vi "GUI_laptop v11f.vi"() -> ()   [LabVIEW 2019]
uses:
  <vilib>/Math Plots/3D Math Plots/3D Scatter/3D Scatter XCtrl/3D Scatter.xctl
  <vilib>/Platform/TimedLoop/XDataNode/timing_clust.ctl
  <vilib>/Platform/TimedLoop/XDataNode/nitl_modes.ctl
  <vilib>/Platform/TimedLoop/XDataNode/wakeup.ctl
  <vilib>/Analysis/_algsub.llb/Real Vector Norm.vi
  <vilib>/Instr/_visa.llb/VISA Configure Serial Port (Instr).vi
  <vilib>/Utility/file.llb/Write Delimited Spreadsheet (DBL).vi
  <vilib>/addons/System Identification/Data Preprocess.llb/SI Lowpass Filter (MISO Array).vi
  <vilib>/Math Plots/3D Math Plots/3D Scatter/3D Scatter Datatype/Public/Plot Helper (Vector).vi
  <vilib>/platform/TimedLoop/XDataNode/XDataNode.xnode
  <vilib>/Platform/TimedLoop/XDataNode/XDNodeRunTimeDep.lvlib
  <vilib>/Analysis/NI_AALPro.lvlib
  <vilib>/Math Plots/3D Math Plots/3D Scatter/3D Scatter Datatype/3D Scatter Datatype.lvclass
  <vilib>/addons/System Identification/NI_SysID.lvlib
panel:
  in  "Sample rate":u32=115200
  in  "Cutoff Frequency":dbl=10.0
  in  "Motion scale L1 L2":dbl=10.0
  in  "Motion scale L3":dbl=2.0
  in  "Save Path 4":path=path "C:/Users/jimmy/Documents/GitHub/Arduino-LabVIEW/zhantao/read_data_abs_filtered.csv"
  in  "Save Path 3":path=path "C:/Users/jimmy/Documents/GitHub/Arduino-LabVIEW/zhantao/read_data_abs_sending.csv"
  out "stimulus signals out":dbl[][](array[numeric]) format="%.2f"
  in  "L5 Offset":dbl
  in  "L5 Scale":dbl=1.0
  in  "Motion Scale L4":dbl=2.0
  out "spreadsheet string":string
  in  "Save Path 2":path=path "C:/Users/jimmy/Documents/GitHub/Arduino-LabVIEW/zhantao/read_data_delt.csv"
  out "send values":dbl[](array[numeric])
  out "Robot Feedback (xyz)":dbl[](array[numeric])
  in  "UDP Send":bool
  in  "UDP Recv":bool
  in  "L5 bound":dbl=1000.0
  in  "L4 bound (deg)":dbl=1000.0
  in  "L3 bound (mm)":dbl=1000.0
  in  "L2 bound (deg)":dbl=1000.0
  in  "L1 bound (deg)":dbl=1000.0
  in  "Joystick Type":dbl(ring) items=["Rigid Joystick", "Free Joystick"]
  out "Finished Late? [i-1]":bool
  in  "Epsilon":dbl=0.2
  out "3D Scatter":refnum<class "3D Plot Datatype.lvclass">[](xcontrol)
  out "Random Point":dbl[](array[numeric])
  out "Virtual Cursor":dbl[](array[numeric])
  out "Iteration Duration":i64
  in  "Num of Points":i32=10
  in  "z bound":dbl=2.0
  in  "y bound":dbl=5.0
  in  "x bound":dbl=5.0
  in  "Stop":bool
  in  "Round Decimals":dbl=2.0 format="%#_15g"
  in  "Save Data":bool
  in  "Save Path":path=path "C:/Users/jimmy/Documents/GitHub/Arduino-LabVIEW/zhantao/read_data_abs.csv"
  in  "x speed":dbl=0.5
  in  "z speed":dbl=0.5
  in  "y speed":dbl=0.5
  out "error out":errorcluster
  in  "baud rate":u32=115200
  in  "VISA resource name":refnum<visa-resource-name>
  # "Joystick Selection"
  # "Plotting"
  # "Data Saving"
  # "Arduino Communication"
  # "Master Slave Communication"
  # "Parameters"
  # "TODO: fix the bounds; currently bounds are arbitrary"
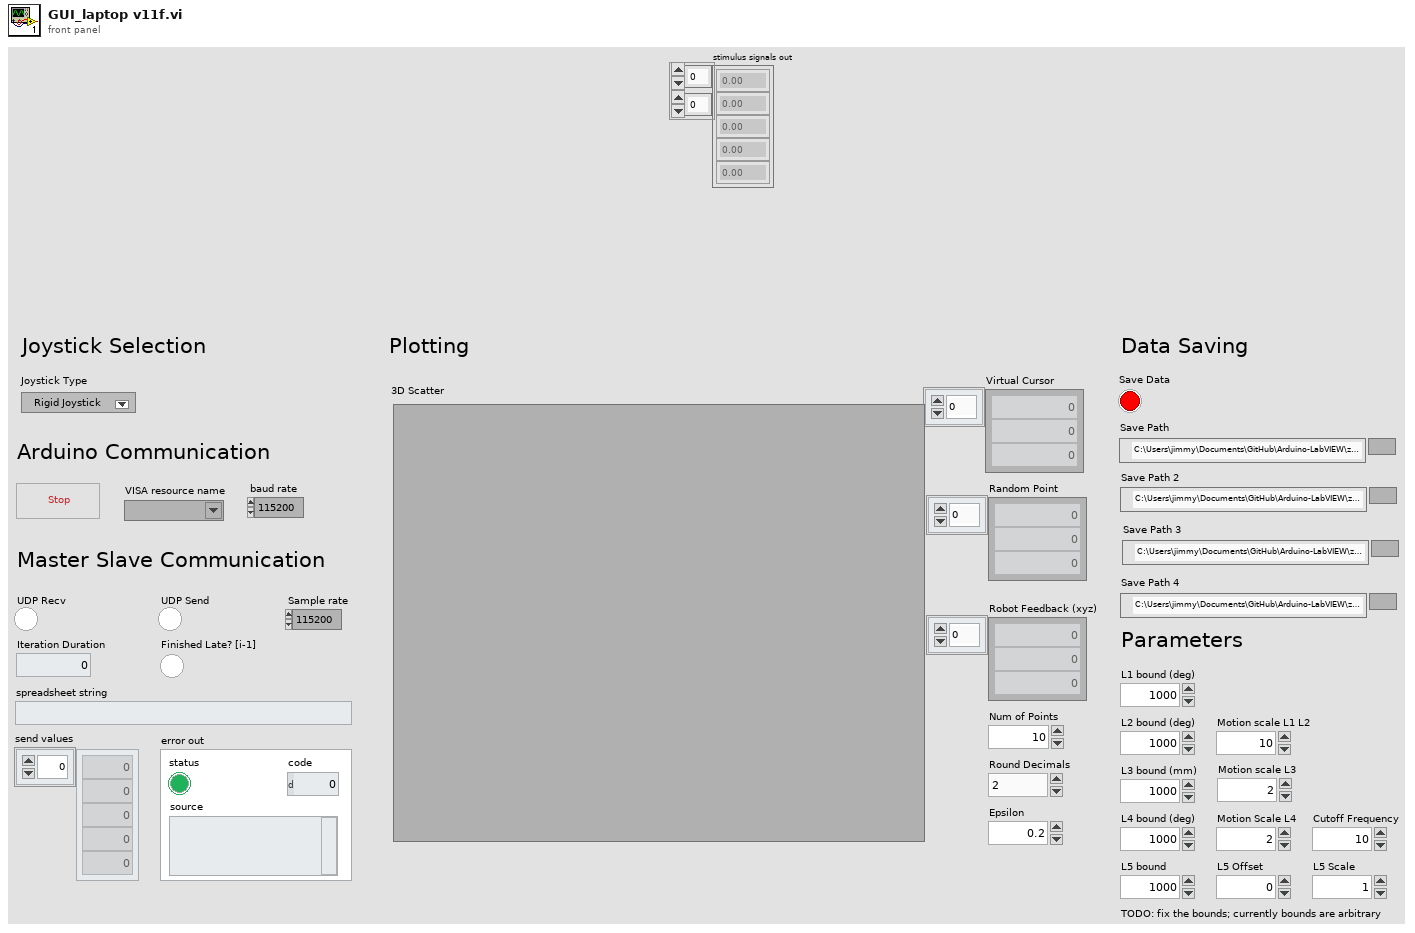
[diagram p1: front panel]
types:
  T1 = typedef "XDNodeRunTimeDep.lvlib/timing_clust.ctl" = cluster{"Expected End [f-1]":u64, "Actual End [f-1]":u64, "Finished Late? [f-1]":bool, "Expected End [i-1]":u64, "Actual End [i-1]":u64, "Finished Late? [i-1]":bool, "Expected Start [i]":u64, "Actual Start [i]":u64, "Expected Start [f]":u64, "Actual Start [f]":u64, "Source Name":string, "Structure Name":string, "Period":i64, "Deadline":i64, "Offset":i64, "Start":i64, "Priority":i32, "Timeout":i32, "Mode":T2, "Wakeup Reason":T3, "Error":errorcluster, "Source Type":string, "Secondary Source Type":string, "Global End Time":u64, "Global Start Time":u64, "Frame Duration":u64, "Iteration Duration":u64, "Assigned CPU":i32, "I/O Scan Engine Mode":u32}
  T2 = typedef "XDNodeRunTimeDep.lvlib/nitl_modes.ctl" = enum32{"No Change", "Process missed periods, maintain original phase", "Discard missed periods, maintain original phase", "Process missed periods, ignore original phase", "Discard missed periods, ignore original phase"}
  T3 = typedef "XDNodeRunTimeDep.lvlib/wakeup.ctl" = enum32{"Normal", "Aborted", "Asynchronous wakeup", "Timing source error", "Timed loop error", "Timeout"}
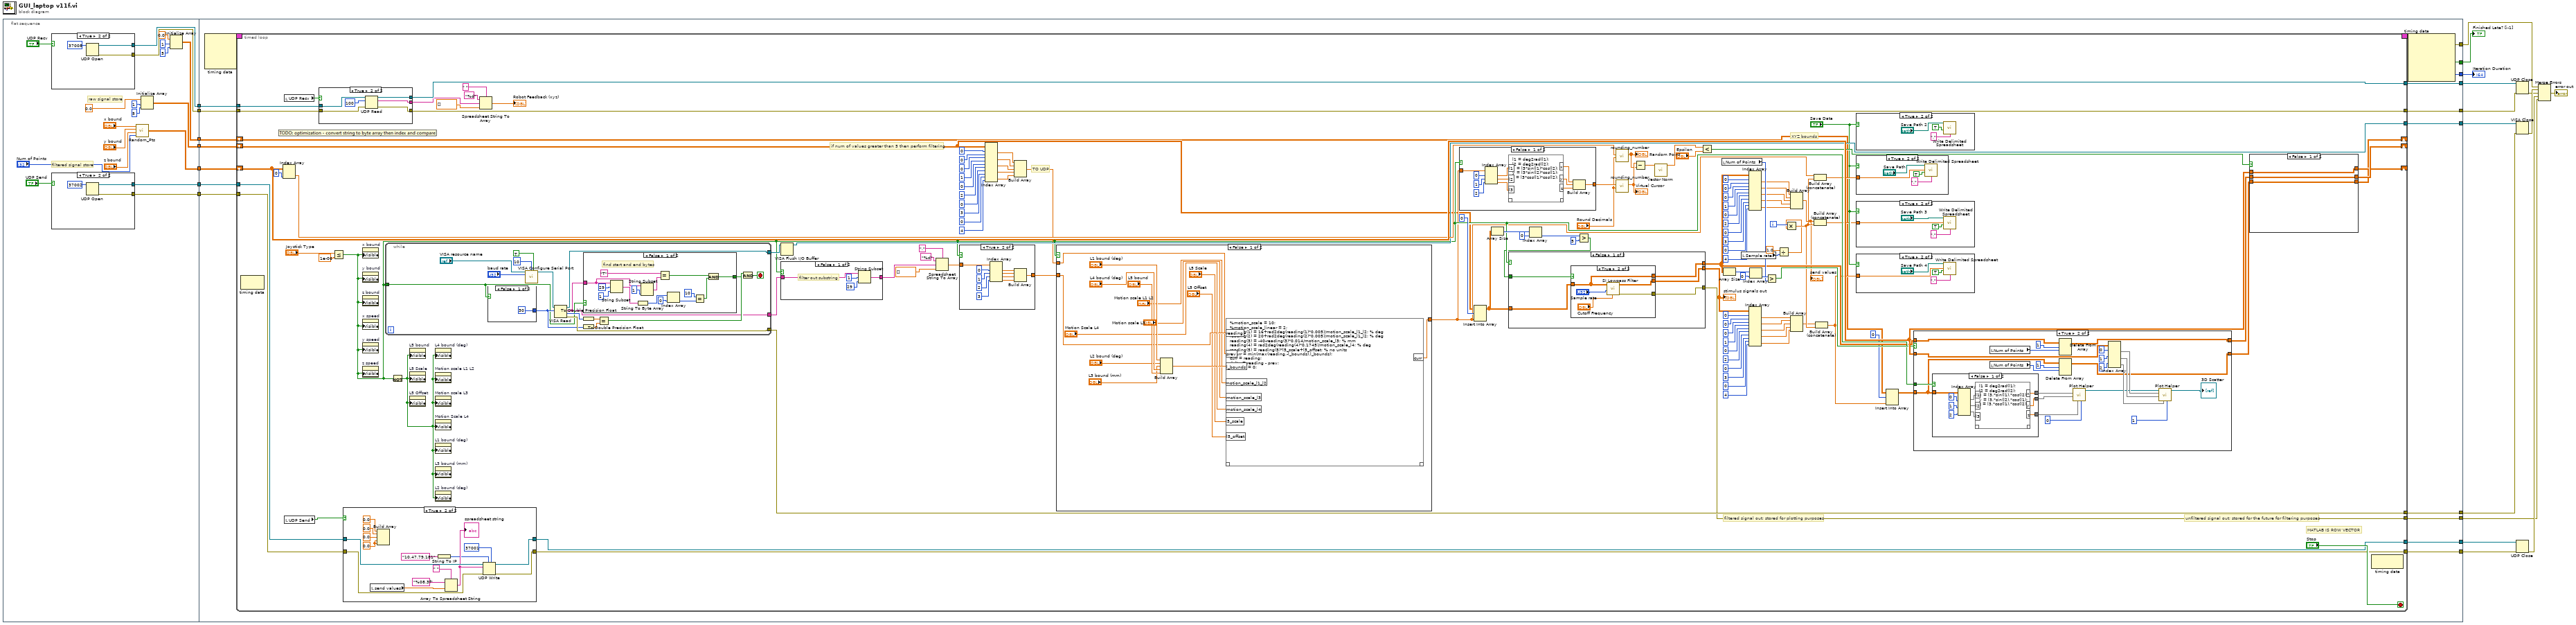
[diagram p0: block diagram]
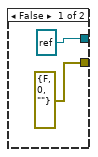
[diagram p2: hidden frame]
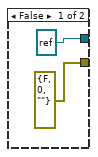
[diagram p3: hidden frame]
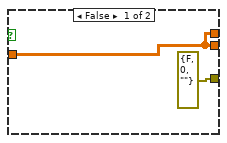
[diagram p6: hidden frame]
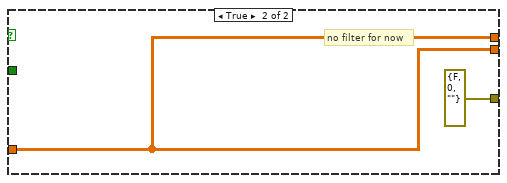
[diagram p7: hidden frame]
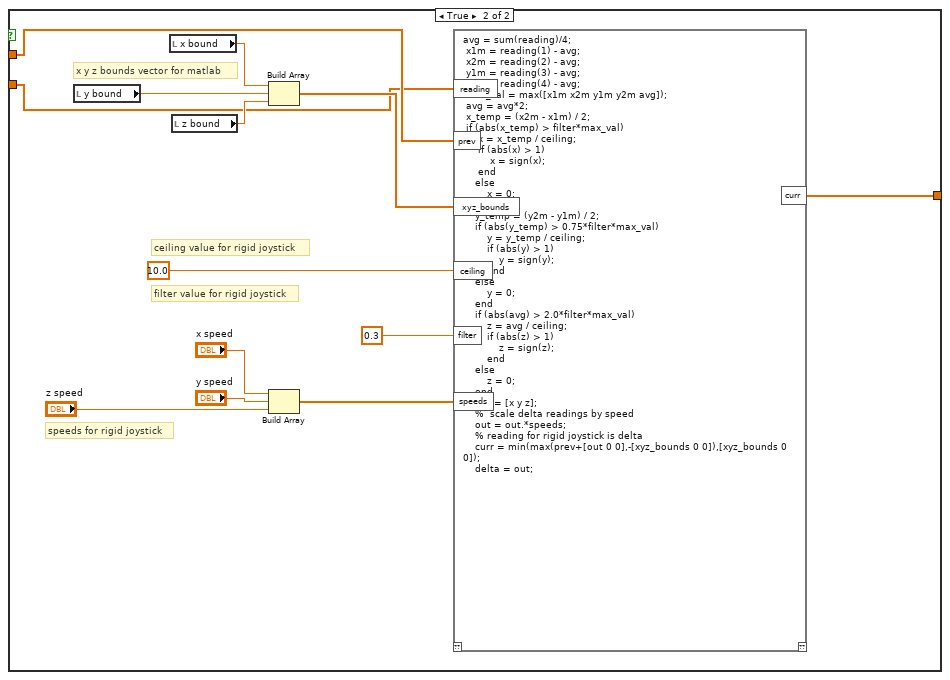
[diagram p8: hidden frame]
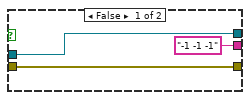
[diagram p11: hidden frame]
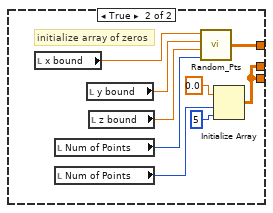
[diagram p13: hidden frame]
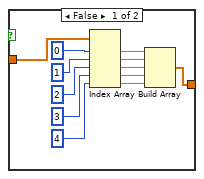
[diagram p15: hidden frame]
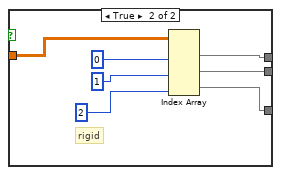
[diagram p18: hidden frame]
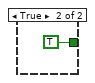
[diagram p19: hidden frame]
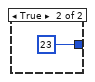
[diagram p20: hidden frame]
diagram:
  n1 = flat-sequence {
    tunnel: [w32] -> w17
    tunnel: [w36] -> w16
    tunnel: [w31] -> w15
    tunnel: [w30] -> w14
    tunnel: [w27] -> w13
    tunnel: [w26] -> w12
    tunnel: [w22] -> w1
    tunnel: [w67] -> w21
    tunnel: [w66] -> w20
    tunnel: [w64] -> w11
    tunnel: [w62] -> w19
    tunnel: [w61] -> w18
    tunnel: w17 -> [w65]
    tunnel: w16 -> [w63]
    tunnel: w15 -> [w60]
    tunnel: w14 -> [w59]
    tunnel: w13 -> [w58]
    tunnel: w12 -> [w57]
    tunnel: [w56] -> w5
    tunnel: [w55] -> w10
    tunnel: [w54] -> w4
    tunnel: [w53] -> w3
    tunnel: [w52] -> w2
    tunnel: w1 -> [w51]
    frame #0 {
      # "filtered signal store"
      # "raw signal store"
      n2 = case shown="True" "UDP Recv" {
        tunnel: [refnum<k16> refnum ("port") w49] -> w30
        tunnel: [errorcluster {"status"=FALSE, "code"=0, "source"=""} ("error out") w48] -> w27
        frame False {
        }
        frame True {
          n3 = UDP Open(11:u16 37008 ("port")) -> (port=w49:refnum<k16>, 0:w48:errorcluster)  [unwired: 4 in, 1 out]
        }
      }
      n4 = case shown="True" "UDP Send" {
        tunnel: [refnum<k16> refnum ("port") w44] -> w31
        tunnel: [errorcluster {"status"=FALSE, "code"=0, "source"=""} ("error out") w43] -> w26
        frame False {
        }
        frame True {
          n5 = UDP Open(11:u16 37002 ("port")) -> (port=w44:refnum<k16>, 0:w43:errorcluster)  [unwired: 4 in, 1 out]
        }
      }
      n6 = call "Random_Pts.vi"("Num of Points"="Num of Points", "z bound"="z bound", "y bound"="y bound", "x bound"="x bound") -> ("appended array"=w36:dbl[][])
      n7 = Initialize Array(0.0 ("element"), 1 ("dimension size"), 5 ("dimension size")) -> (w32:dbl[][])
      n8 = Initialize Array(0.0 ("element"), 1 ("dimension size"), 5 ("dimension size")) -> (w22:dbl[][])
    }
    frame #1 {
      n9 = node-c288() -> (w69:T1)  [unwired: 4 in]
      n10 = timed-loop {
        tunnel: [w134] -> w67
        tunnel: [w191] -> w66
        shift-right: [w190] -> _
        shift-left: w65 -> [w88]
        timing: w69 -> [_]
        timing-out: [_] -> w68
        shift-right: [w186] -> _
        shift-left: w63 -> [w187]
        tunnel: w60 -> [w149]
        tunnel: w59 -> [w148]
        tunnel: w58 -> [w146]
        tunnel: w57 -> [w145]
        tunnel: [w144] -> w56
        tunnel: [w143] -> w55
        tunnel: [w142] -> w54
        tunnel: [w141] -> w53
        tunnel: [w123] -> w52
        shift-right: [w79] -> _
        shift-left: w51 -> [w82]
        i -> [w77]
        stop <- "Stop" stop-if-true
        # "unfiltered signal out; stored for the future for filtering purposes"
        # "filtered signal out; stored for plotting purposes"
        # "XYZ bounds"
        # "if num of values greater than 5 then perform filtering"
        # "TO UDP"
        # "MATLAB IS ROW VECTOR"
        n11 = node-c288() -> ()  [unwired: 1 in, 1 out]
        n12 = Index Array(array=w187, index (col)=0 ("index (row)")) -> (element=w158:dbl[])  [unwired: 1 in]
        n13 = local read "UDP Recv"() -> (w147:bool)
        n14 = local read "UDP Send"() -> (w72:bool)
        n15 = case shown="True" w147 {
          tunnel: w148 -> [w263 w270]
          tunnel: w146 -> [w264 w269]
          tunnel: [w264 w268] -> w144
          tunnel: [w263 w267] -> w142
          tunnel: ["-1 -1 -1" w265] -> w137
          frame False {
          }
          frame True {
            n16 = UDP Read(connection ID=w270, max size (548)=100, 8:w269) -> (data out=w265:string, error out=w268:errorcluster, 3:w267:refnum<k16>)  [unwired: 1 in, 2 out]
          }
        }
        n17 = Less Or Equal?(x="Joystick Type", y=1e-06) -> (x <= y?=w124:bool)
        n18 = case shown="True" w72 {
          tunnel: w149 -> [w245 w261]
          tunnel: w145 -> [w246 w257]
          tunnel: [w246 w253] -> w143
          tunnel: [w245 w252] -> w141
          frame False {
          }
          frame True {
            w251 = 0.0 ("element")
            n19 = local read "send values"() -> (w247:dbl[])
            n20 = Build Array(0.0 ("element"), 0.0 ("element"), 0.0 ("element"), w251, w251) -> ()  [unwired: 1 out]
            n21 = String To IP(1:"10.47.79.181" ("name")) -> (0:w255:u32)
            n22 = Array To Spreadsheet String(delimiter (Tab)=" ", array=w247, 3:"%08.3f" ("format string")) -> (spreadsheet string=w258:string)
            "spreadsheet string" <- w258
            n23 = UDP Write(address=w255, port or service name=u16 37001, connection ID=w261, data in=w258, 8:w257) -> (error out=w253:errorcluster, 3:w252:refnum<k16>)  [unwired: 1 in]
          }
        }
        n24 = property on="x bound" class="DigNum (strict)"("Visible"=w124) -> ()  [unwired: 2 in, 2 out]
        n25 = property on="y bound" class="DigNum (strict)"("Visible"=w124) -> ()  [unwired: 2 in, 2 out]
        n26 = property on="z bound" class="DigNum (strict)"("Visible"=w124) -> ()  [unwired: 2 in, 2 out]
        n27 = property on="x speed" class="DigNum (strict)"("Visible"=w124) -> ()  [unwired: 2 in, 2 out]
        n28 = property on="y speed" class="DigNum (strict)"("Visible"=w124) -> ()  [unwired: 2 in, 2 out]
        n29 = property on="z speed" class="DigNum (strict)"("Visible"=w124) -> ()  [unwired: 2 in, 2 out]
        n30 = while {
          tunnel: [w368] -> w160
          tunnel: [w381] -> w191
          tunnel: [w375] -> w135
          tunnel: w124 -> [w369]
          stop <- w371 stop-if-true
          n31 = case shown="False" w369 {
            tunnel: [30 u32 23 ("byte count")] -> w374
            frame False {
            }
            frame True {
            }
          }
          n32 = call-poly "VISA Configure Serial Port"("VISA resource name"="VISA resource name", "termination char\n(0xA = '\\n' = LF)"=u8 10 ("termination char\n(0xA = '\\n' = LF)"), "Enable Termination\nChar (T)"=TRUE ("Enable Termination\nChar (T)"), "baud rate (9600)"="baud rate") -> ("VISA resource name out"=w376:refnum<visa-resource-name>)  [unwired: 10 in, 1 out]
          n33 = VISA Read(VISA resource name=w376, byte count=w374) -> (VISA resource name out=w375:refnum<visa-resource-name>, read buffer=w368:string, return count=w383:u32, error out=w381:errorcluster)  [unwired: 1 in]
          n34 = To Double Precision Float(number=w383) -> (double precision float=w382:dbl)
          n35 = To Double Precision Float(number=w374) -> (double precision float=w373:dbl)
          n36 = case shown="False" w369 {
            tunnel: [w390 TRUE] -> w370
            tunnel: w368 -> [w393 _]
            frame False {
              # "find start and end bytes"
              n37 = String Subset(string=w393, offset (0)=29, length (rest)=1) -> (substring=w388:string)
              n38 = String To Byte Array(string=w388) -> (unsigned byte array=w387:u8[])
              n39 = String Subset(string=w393, length (rest)=1) -> (substring=w396:string)  [unwired: 1 in]
              n40 = Equal?(x="T", y=w396) -> (x = y?=w392:bool)
              n41 = Index Array(array=w387, index=0) -> (element=w385:u8)
              n42 = Equal?(x=10, y=w385) -> (x = y?=w391:bool)
              n43 = And(x=w392, y=w391) -> (x .and. y?=w390:bool)
            }
            frame True {
            }
          }
          n44 = Equal?(x=w382, y=w373) -> (x = y?=w372:bool)
          n45 = And(x=w372, y=w370) -> (x .and. y?=w371:bool)
        }
        n46 = Not(x=w124) -> (.not. x?=w86:bool)
        n47 = property on="L5 bound" class="DigNum (strict)"("Visible"=w86) -> ()  [unwired: 2 in, 2 out]
        n48 = property on="L5 Scale" class="DigNum (strict)"("Visible"=w86) -> ()  [unwired: 2 in, 2 out]
        n49 = property on="L5 Offset" class="DigNum (strict)"("Visible"=w86) -> ()  [unwired: 2 in, 2 out]
        n50 = property on="L4 bound (deg)" class="DigNum (strict)"("Visible"=w86) -> ()  [unwired: 2 in, 2 out]
        n51 = property on="Motion scale L1 L2" class="DigNum (strict)"("Visible"=w86) -> ()  [unwired: 2 in, 2 out]
        n52 = property on="Motion scale L3" class="DigNum (strict)"("Visible"=w86) -> ()  [unwired: 2 in, 2 out]
        n53 = property on="Motion Scale L4" class="DigNum (strict)"("Visible"=w86) -> ()  [unwired: 2 in, 2 out]
        n54 = property on="L1 bound (deg)" class="DigNum (strict)"("Visible"=w86) -> ()  [unwired: 2 in, 2 out]
        n55 = property on="L3 bound (mm)" class="DigNum (strict)"("Visible"=w86) -> ()  [unwired: 2 in, 2 out]
        n56 = property on="L2 bound (deg)" class="DigNum (strict)"("Visible"=w86) -> ()  [unwired: 2 in, 2 out]
        n57 = Spreadsheet String To Array(delimiter (Tab)=" ", format string="%d", spreadsheet string=w137, array type (2D Dbl)=dbl[] []) -> (array=→"Robot Feedback (xyz)":dbl[])
        n58 = VISA Flush I/O Buffer(VISA resource name=w135) -> (VISA resource name out=w134:refnum<visa-resource-name>)  [unwired: 2 in, 1 out]
        n59 = case shown="False" w124 {
          tunnel: w160 -> [w290 w291]
          tunnel: [w287 w291] -> w159
          frame False {
            # "filter out substring"
            n60 = String Subset(string=w290, offset (0)=1, length (rest)=29) -> (substring=w287:string)
          }
          frame True {
          }
        }
        n61 = Spreadsheet String To Array(delimiter (Tab)=",", format string="%d", spreadsheet string=w159, array type (2D Dbl)=dbl[] []) -> (array=w161:dbl[])
        n62 = case shown="True" w124 {
          tunnel: w161 -> [w292 w307]
          tunnel: [w297 w306] -> w132
          frame False {
            n63 = Index Array(array=w292, index #1=0 ("Plot ID"), index #2=1 ("Plot ID"), index #3=2 ("Plot ID"), index #4=3 ("Plot ID"), index #5=4 ("Plot ID")) -> (element #1=w300:dbl, element #2=w299:dbl, element #3=w298:dbl, element #4=w294:dbl, element #5=w293:dbl)
            n64 = Build Array(w300, w299, w298, w294, w293) -> (w297:dbl[])
          }
          frame True {
            n65 = Index Array(array=w307, index #1=0 ("Plot ID"), index #2=1 ("Plot ID"), index #3=2 ("Plot ID"), index #4=3 ("index")) -> (element #1=w310:dbl, element #2=w309:dbl, element #3=w308:dbl, element #4=w304:dbl)
            n66 = Build Array(w310, w309, w308, w304) -> (w306:dbl[])
          }
        }
        n67 = Index Array(array=w88, index (row) #1=0 ("disabled index (row)"), index (col) #1=0 ("disabled index (col)"), index (row) #2=0 ("disabled index (row)"), index (col) #2=1 ("disabled index (col)"), index (row) #3=0 ("disabled index (row)"), index (col) #3=2 ("disabled index (col)"), index (row) #4=0 ("disabled index (row)"), index (col) #4=3 ("disabled index (col)"), index (row) #5=0 ("disabled index (row)"), index (col) #5=4 ("disabled index (col)")) -> (element #1=w172:dbl, element #2=w171:dbl, element #3=w170:dbl, element #4=w163:dbl, element #5=w162:dbl)
        n68 = Build Array(w172, w171, w170, w163, w162) -> (w133:dbl[])
        n69 = case shown="False" w124 {
          tunnel: w133 -> [w220 w231]
          tunnel: w132 -> [w221 w230]
          tunnel: [w219 w229] -> w107
          frame False {
            n70 = Build Array("L1 bound (deg)", "L2 bound (deg)", "L3 bound (mm)", "L4 bound (deg)", "L5 bound") -> (w222:dbl[])
            n71 = script code="%motion_scale = 10;\n%motion_scale_linear = 2;\nreading(1) = 16+rad2deg(reading(1)*0.005)/motion_scale_l1_l2; % deg\nreading(2) = 20+rad2deg(reading(2)*0.005)/motion_scale_l1_l2; % deg\nreading(3) = -40-reading(3)*0.014/motion_scale_l3; % mm\nreading(4) = rad2deg(reading(4)*0.1745)/motion_scale_l4; % deg\nreading(5) = reading(5)*l5_scale+l5_offset; % no units\n%curr = min(max(reading,-l_bounds),l_bounds);\ncurr = reading;\ndelta = reading - prev;\ndelta(5) = 0;"("l_bounds"=w222, "motion_scale_l4"="Motion Scale L4", "reading"=w221, "prev"=w220, "l5_scale"="L5 Scale", "l5_offset"="L5 Offset", "motion_scale_l3"="Motion scale L3", "motion_scale_l1_l2"="Motion scale L1 L2") -> ("curr"=w219:dbl[])  [unwired: 1 in, 1 out]
          }
          frame True {
            # "ceiling value for rigid joystick"
            # "filter value for rigid joystick"
            # "speeds for rigid joystick"
            # "x y z bounds vector for matlab"
            n72 = local read "y bound"() -> (w240:dbl)
            n73 = local read "x bound"() -> (w239:dbl)
            n74 = local read "z bound"() -> (w241:dbl)
            n75 = Build Array(w239, w240, w241) -> (w232:dbl[])
            n76 = Build Array("x speed", "y speed", "z speed") -> (w235:dbl[])
            n77 = script code="avg = sum(reading)/4;\n x1m = reading(1) - avg;\n x2m = reading(2) - avg;\n y1m = reading(3) - avg;\n y2m = reading(4) - avg;\n max_val = max([x1m x2m y1m y2m avg]);\n avg = avg*2;\n x_temp = (x2m - x1m) / 2;\n if (abs(x_temp) > filter*max_val)\n     x = x_temp / ceiling;\n     if (abs(x) > 1)\n         x = sign(x);\n     end\n    else\n        x = 0;\n    end\n    y_temp = (y2m - y1m) / 2;\n    if (abs(y_temp) > 0.75*filter*max_val)\n        y = y_temp / ceiling;\n        if (abs(y) > 1)\n            y = sign(y);\n        end\n    else\n        y = 0;\n    end\n    if (abs(avg) > 2.0*filter*max_val)\n        z = avg / ceiling;\n        if (abs(z) > 1)\n            z = sign(z);\n        end\n    else\n        z = 0;\n    end\n    out = [x y z];\n    %  scale delta readings by speed\n    out = out.*speeds;\n    % reading for rigid joystick is delta\n    curr = min(max(prev+[out 0 0],-[xyz_bounds 0 0]),[xyz_bounds 0 0]);\n    delta = out;"("xyz_bounds"=w232, "ceiling"=10.0 ("Real"), "filter"=0.3 ("Real"), "speeds"=w235, "reading"=w230, "prev"=w231) -> ("curr"=w229:dbl[])  [unwired: 1 in, 1 out]
          }
        }
        n78 = case shown="False" w124 {
          tunnel: [w318 w325] -> w188
          tunnel: w107 -> [w317 w325]
          frame False {
            n79 = Index Array(array=w317, index #1=0 ("Plot ID"), index #2=1 ("Plot ID"), index #3=2 ("Plot ID")) -> (element #1=w316:dbl, element #2=w315:dbl, element #3=w314:dbl)
            n80 = script code="l1 = deg2rad(l1);\nl2 = deg2rad(l2);\nx = l3*sin(l1)*cos(l2);\ny = l3*sin(l2)*cos(l1);\nz = l3*cos(l1)*cos(l2);"("l1"=w316, "l2"=w315, "l3"=w314) -> ("x"=w321:dbl, "y"=w320:dbl, "z"=w319:dbl)  [unwired: 1 in, 1 out]
            n81 = Build Array(w321, w320, w319) -> (w318:dbl[])
          }
          frame True {
          }
        }
        n82 = Insert Into Array(array=w88, index (row)=0, new element=w107) -> (w125:dbl[][])  [unwired: 1 in]
        n83 = Array Size(array=w125) -> (size(s)=w128:i32[])
        n84 = Index Array(array=w128, index=0) -> (element=w127:i32)
        n85 = Greater?(x=w127, y=5) -> (0:w73:bool)
        n86 = case shown="False" w124 {
          tunnel: w73 -> [w203 _]
          tunnel: w125 -> [w205 w213]
          tunnel: [w204 w213] -> w85
          tunnel: [w202 errorcluster {"status"=FALSE, "code"=0, "source"=""} ("error out")] -> w123
          tunnel: [w201 w213] -> w89
          frame False {
            n87 = case shown="True" w203 {
              tunnel: w205 -> [w206 w211]
              tunnel: [w206 w211] -> w204
              tunnel: [errorcluster {"status"=FALSE, "code"=0, "source"=""} ("error out") w212] -> w202
              tunnel: [w206 w210] -> w201
              frame False {
              }
              frame True {
                n88 = call-poly <vilib>:"SI Lowpass Filter.vi"("cutoff frequency"="Cutoff Frequency", "sampling rate (Hz)"="Sample rate", "stimulus signals in"=w211) -> ("error out"=w212:errorcluster, "stimulus signals out"=w210:dbl[][])  [unwired: 6 in, 1 out]
              }
            }
          }
          frame True {
            # "no filter for now"
          }
        }
        "stimulus signals out" <- w89
        n89 = call "rounding_number.vi"("power of ten"="Round Decimals", "Array"=w158) -> ("rounded"=w155:dbl[])  [unwired: 9 in]
        "Random Point" <- w155
        n90 = call "rounding_number.vi"("power of ten"="Round Decimals", "Array"=w188) -> ("rounded"=w156:dbl[])  [unwired: 9 in]
        "Virtual Cursor" <- w156
        n91 = Subtract(x=w156, y=w155) -> (x-y=w154:dbl[])
        n92 = call-poly <vilib>:"Vector Norm.vi"("Input Vector"=w154) -> ("norm"=w153:dbl)  [unwired: 9 in, 1 out]
        n93 = Less?(x=w153, y="Epsilon") -> (x < y?=w151:bool)
        n94 = local read "Num of Points"() -> (w174:i32)
        n95 = Array Size(array=w85) -> (size(s)=w131:i32[])
        n96 = local read "Sample rate"() -> (w74:u32)
        n97 = Index Array(array=w85, index (row) #1=0 ("disabled index (col)"), index (col) #1=0 ("disabled index (row)"), index (row) #2=0 ("disabled index (col)"), index (col) #2=1 ("disabled index (row)"), index (row) #3=0 ("disabled index (col)"), index (col) #3=2 ("disabled index (row)"), index (row) #4=0 ("disabled index (col)"), index (col) #4=3 ("disabled index (row)"), index (row) #5=0 ("disabled index (col)"), index (col) #5=4 ("disabled index (col)")) -> (element #1=w112:dbl, element #2=w111:dbl, element #3=w110:dbl, element #4=w109:dbl, element #5=w108:dbl)
        n98 = Index Array(array=w89, index (row) #1=0 ("disabled index (col)"), index (col) #1=0 ("disabled index (row)"), index (row) #2=0 ("disabled index (col)"), index (col) #2=1 ("disabled index (row)"), index (row) #3=0 ("disabled index (col)"), index (col) #3=2 ("disabled index (row)"), index (row) #4=0 ("disabled index (col)"), index (col) #4=3 ("disabled index (row)"), index (row) #5=0 ("disabled index (col)"), index (col) #5=4 ("disabled index (col)")) -> (element #1=w95:dbl, element #2=w94:dbl, element #3=w93:dbl, element #4=w92:dbl, element #5=w91:dbl)
        n99 = Index Array(array=w131, index=0) -> (element=w175:i32)
        n100 = Greater?(x=w175, y=w174) -> (0:w173:bool)
        n101 = Divide(x=1.0, y=w74) -> (x/y=w75:dbl)
        n102 = Multiply(x=w77, y=w75) -> (x*y=w78:dbl)
        n103 = Build Array(w112, w111, w110, w109, w108) -> (w70:dbl[])
        "send values" <- w70
        n104 = Build Array(w95, w94, w93, w92, w91) -> (w71:dbl[])
        n105 = Build Array (concatenate)(w107, w78) -> (w106:dbl[])
        n106 = Build Array (concatenate)(w70, w78) -> (w87:dbl[])
        n107 = Build Array (concatenate)(w71, w78) -> (w83:dbl[])
        n108 = case shown="True" "Save Data" {
          frame False {
          }
          frame True {
            n109 = call-poly <vilib>:"Write Delimited Spreadsheet.vi"("file path (dialog if empty)"="Save Path 2", "append to file? (new file:F)"=TRUE, "delimiter (\\t)"="," ("delimiter (\\t)")) -> ()  [unwired: 11 in, 2 out]
          }
        }
        n110 = case shown="True" "Save Data" {
          tunnel: w106 -> [_ w271]
          frame False {
          }
          frame True {
            n111 = call-poly <vilib>:"Write Delimited Spreadsheet.vi"("file path (dialog if empty)"="Save Path", "1D data"=w271, "append to file? (new file:F)"=TRUE, "delimiter (\\t)"="," ("delimiter (\\t)")) -> ()  [unwired: 10 in, 2 out]
          }
        }
        n112 = case shown="True" "Save Data" {
          tunnel: w87 -> [_ w197]
          frame False {
          }
          frame True {
            n113 = call-poly <vilib>:"Write Delimited Spreadsheet.vi"("file path (dialog if empty)"="Save Path 3", "1D data"=w197, "append to file? (new file:F)"=TRUE, "delimiter (\\t)"="," ("delimiter (\\t)")) -> ()  [unwired: 10 in, 2 out]
          }
        }
        n114 = case shown="True" "Save Data" {
          tunnel: w83 -> [_ w193]
          frame False {
          }
          frame True {
            n115 = call-poly <vilib>:"Write Delimited Spreadsheet.vi"("file path (dialog if empty)"="Save Path 4", "1D data"=w193, "append to file? (new file:F)"=TRUE, "delimiter (\\t)"="," ("delimiter (\\t)")) -> ()  [unwired: 10 in, 2 out]
          }
        }
        n116 = Insert Into Array(array=w82, index (row)=0, new element=w83) -> (w81:dbl[][])  [unwired: 1 in]
        n117 = case shown="True" w173 {
          tunnel: w85 -> [w327 w349]
          tunnel: [w327 w348] -> w189
          tunnel: w187 -> [w326 w347]
          tunnel: w124 -> [_ w332]
          tunnel: w81 -> [_ w329]
          tunnel: [w326 w328] -> w80
          frame False {
          }
          frame True {
            n118 = case shown="False" w332 {
              tunnel: w329 -> [w360 w364]
              tunnel: [w351 w363] -> w338
              tunnel: [w352 w362] -> w337
              tunnel: [w353 w361] -> w336
              frame False {
                n119 = Index Array(array=w360, index (col) #1=0 ("Plot ID"), index (col) #2=1 ("Plot ID"), index (col) #3=2 ("Plot ID")) -> (element #1=w356:dbl[], element #2=w355:dbl[], element #3=w354:dbl[])  [unwired: 3 in]
                n120 = script code="l1 = deg2rad(l1);\nl2 = deg2rad(l2);\nx = l3.*sin(l1).*cos(l2);\ny = l3.*sin(l2).*cos(l1);\nz = l3.*cos(l1).*cos(l2);"("l1"=w356, "l2"=w355, "l3"=w354) -> ("x"=w351:dbl[], "y"=w352:dbl[], "z"=w353:dbl[])  [unwired: 1 in, 1 out]
              }
              frame True {
                # "rigid"
                n121 = Index Array(array=w364, index (col) #1=0 ("disabled index (col)"), index (col) #2=1 ("index (col)"), index (col) #3=2 ("index (col)")) -> (element #1=w363:dbl[], element #2=w362:dbl[], element #3=w361:dbl[])  [unwired: 3 in]
              }
            }
            n122 = local read "Num of Points"() -> (w346:i32)
            n123 = local read "Num of Points"() -> (w331:i32)
            n124 = Delete From Array(array=w349, length=1, index (row)=w346) -> (array with subset deleted=w348:dbl[][])  [unwired: 1 in, 1 out]
            n125 = Delete From Array(array=w329, length=1, index (row)=w331) -> (array with subset deleted=w328:dbl[][])  [unwired: 1 in, 1 out]
            n126 = call-poly <vilib>:"Plot Helper.vi"("Plot ID"=0, "z vector"=w336, "y vector"=w337, "x vector"=w338) -> ("3D Plot lvclass Array out"=w340:refnum<class "3D Plot Datatype.lvclass">[])  [unwired: 2 in, 5 out]
            n127 = Index Array(array=w347, index (row) #1=0 ("index (row)"), index (row) #2=1 ("index (row)"), index (row) #3=2 ("index (row)")) -> (element #1=w344:dbl[], element #2=w343:dbl[], element #3=w342:dbl[])  [unwired: 3 in]
            n128 = call-poly <vilib>:"Plot Helper.vi"("Plot ID"=1, "z vector"=w342, "y vector"=w343, "x vector"=w344, "3D Plot lvclass Array in"=w340) -> ("3D Plot lvclass Array out"=→"3D Scatter":refnum<class "3D Plot Datatype.lvclass">[])  [unwired: 1 in, 5 out]
          }
        }
        n129 = case shown="False" w151 {
          tunnel: w187 -> [w277 _]
          tunnel: [w277 w282] -> w186
          tunnel: w189 -> [w276 _]
          tunnel: [w276 w278] -> w190
          tunnel: w80 -> [w275 _]
          tunnel: [w275 w278] -> w79
          frame False {
          }
          frame True {
            # "initialize array of zeros"
            n130 = local read "x bound"() -> (w286:dbl)
            n131 = local read "Num of Points"() -> (w283:i32)
            n132 = local read "Num of Points"() -> (w280:i32)
            n133 = local read "y bound"() -> (w285:dbl)
            n134 = local read "z bound"() -> (w284:dbl)
            n135 = call "Random_Pts.vi"("Num of Points"=w283, "z bound"=w284, "y bound"=w285, "x bound"=w286) -> ("appended array"=w282:dbl[][])
            n136 = Initialize Array(0.0 ("element"), w280, 5 ("dimension size")) -> (w278:dbl[][])
          }
        }
        n137 = node-c288() -> ()  [unwired: 1 in, 1 out]
      }
      n138 = node-c288(w68) -> (w64:errorcluster, w61:bool, w62:i64)  [unwired: 3 out]
    }
  }
  n139 = UDP Close(connection ID=w4, 8:w5) -> (error out=w8:errorcluster)  [unwired: 1 out]
  n140 = VISA Close(VISA resource name=w21, error in (no error)=w20) -> (error out=w9:errorcluster)
  n141 = UDP Close(connection ID=w3, 8:w10) -> (error out=w7:errorcluster)  [unwired: 1 out]
  n142 = Merge Errors(w11, w9, w8, w7, w2) -> (→"error out":errorcluster)
  "Iteration Duration" <- w19
  "Finished Late? [i-1]" <- w18
